vi "datasocket_read.vi"(11 "URL":string) -> (0 "error out":errorcluster caption="错误输出")   [LabVIEW 2018]
uses:
  variable/weatherdata.vi
  variable/stop.vi
panel:
  in  "stop":bool caption="停止"
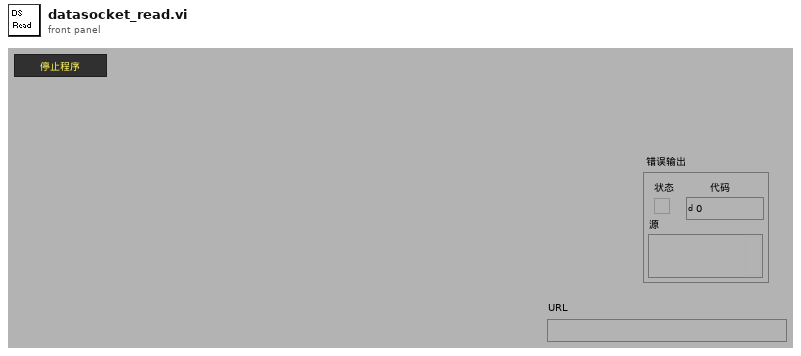
[diagram p1: front panel]
types:
  T1 = enum32{"Reserved1", "Reserved2", "Read", "ReadAutoUpdate", "Write", "WriteAutoUpdate"}
  T2 = typedef "DataSocket Reference Type.ctl" = cluster{"CWDSLib._DCWDataSocket":refnum<k7>, "CWDSLib._DCWData":refnum<k7>, "OnDataUpdated":u32, "OnStatusUpdated":u32}
  T3 = cluster{"温度":dbl, "降雨量":dbl, "风向":dbl, "相对湿度":dbl, "气压":dbl, "风速":dbl, "日期":string, "时间":string}[]
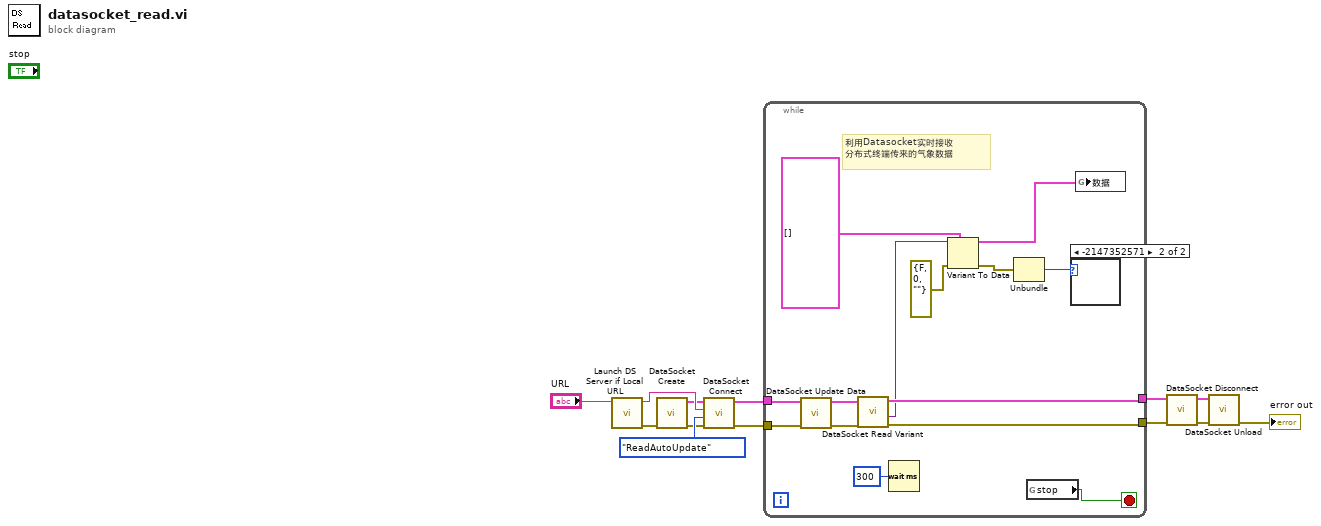
[diagram p0: block diagram]
diagram:
  n1 = call <vilib>:"Launch DS Server if Local URL.vi"("URL"="URL") -> ("error out"=w10:errorcluster, "Duplicate URL"=w12:string)  [unwired: 5 in]
  n2 = call <vilib>:"DataSocket Create.vi"("error in (no error)"=w10) -> ("error out"=w9:errorcluster, "DataSocket Reference Out"=w11:T2)  [unwired: 7 in]
  n3 = call <vilib>:"DataSocket Connect.vi"("error in (no error)"=w9, "AccessMode (ReadAutoUpdate)"=T1."ReadAutoUpdate", "URL"=w12, "DataSocket Reference In"=w11) -> ("error out"=w7:errorcluster, "DataSocket Reference Out"=w8:T2)  [unwired: 4 in]
  n4 = while {
    tunnel: w8 -> [w27]
    tunnel: w7 -> [w26]
    tunnel: [w25] -> w6
    tunnel: [w24] -> w3
    stop <- w15 stop-if-true
    # "利用Datasocket实时接收\n分布式终端传来的气象数据"
    n5 = call <vilib>:"DataSocket Update Data.vi"("Error in (no error)"=w26, "DataSocket Reference In"=w27) -> ("Error out"=w23:errorcluster, "DataSocket Reference Out"=w22:T2)  [unwired: 6 in]
    n6 = call <vilib>:"DataSocket Read Variant.vi"("error in (no error)"=w23, "DataSocket Reference In"=w22) -> ("error out"=w24:errorcluster, "Data"=w21:variant, "DataSocket Reference Out"=w25:T2)  [unwired: 3 in, 2 out]
    n7 = Wait (ms)(milliseconds to wait=u32 300 ("等待时间（毫秒）")) -> ()  [unwired: 1 out]
    n8 = Variant To Data(error in=errorcluster {"status"=FALSE, "code"=0, "source"=""} ("错误输入"), type=T3 [] ("添加的数组"), Variant=w21) -> (data=w16:T3, error out=w18:errorcluster)
    n9 = Unbundle(w18) -> ("code"=w17:i32)  [unwired: 2 out]
    n10 = global read "stop.vi" "stop"() -> (w15:bool)
    n11 = case shown="-2147352571" w17 {
      frame 0, Default {
      }
      frame -2147352571 {
      }
    }
    n12 = global write "weatherdata.vi" "数据"(w16) -> ()
  }
  n13 = call <vilib>:"DataSocket Disconnect.vi"("error in (no error)"=w3, "DataSocket Reference In"=w6) -> ("error out"=w4:errorcluster, "DataSocket Reference Out"=w5:T2)  [unwired: 6 in]
  n14 = call <vilib>:"DataSocket Unload.vi"("error in (no error)"=w4, "DataSocket Reference In"=w5) -> ("error out"=→"error out":errorcluster)  [unwired: 7 in]
